vi "ROTPEN Model Validation.vi"() -> ()   [LabVIEW 2018]
uses:
  <vilib>/Simulation/Scripting/Companion Diagram/SimConfigNode/SimParams.ctl
  <vilib>/Simulation/Scripting/Companion Diagram/SimConfigNode/_simSolvers.ctl
  <vilib>/Simulation/Implementation/Shared/SIMSCR Execution Mode.ctl
  <vilib>/Platform/TimedLoop/XDataNode/timing_clust.ctl
  <vilib>/Platform/TimedLoop/XDataNode/nitl_modes.ctl
  <vilib>/Platform/TimedLoop/XDataNode/wakeup.ctl
  <vilib>/Simulation/Param Hierarchy/Typedefs/SIMPH Param Control Actions.ctl
  <vilib>/Simulation/Scripting/Editor Utilities/SIM subVI tag data.ctl
  <vilib>/Simulation/Scripting/Editor Utilities/SIM subVI execution type.ctl
  <vilib>/Simulation/Implementation/Shared/NILVSim_ParamChanged.vi
  <vilib>/Simulation/Implementation/Shared/NILVSim_FinishedLate.vi
  <vilib>/Simulation/Implementation/Shared/NILVSIM_BeginStep.vi
  <vilib>/Simulation/Utility/Implementation/SIM Halt.vi
  <vilib>/Simulation/SignalArithmetic/Implementation/NILVSim Gain.llb/SIM Gain (scalar).vi
  <vilib>/Simulation/ContinuousLinear/Implementation/NILVSim Derivative.llb/SIM derivative (scalar).vi
  <vilib>/Simulation/ContinuousLinear/Implementation/NILVSim Transfer Function.llb/SIM Transfer Function Distributor (SISO).vi
  <vilib>/Simulation/ContinuousLinear/Implementation/NILVSim Transfer Function.llb/SIM Transfer Function Collector (SISO).vi
  <vilib>/Simulation/Implementation/Shared/SIM Fire Discrete SubVI.vi
  <vilib>/Simulation/Implementation/Shared/NILVSim_Manager.vi
  <vilib>/Utility/error.llb/Clear Errors.vi
  <vilib>/Simulation/Implementation/Shared/NILVSim_FinalizeModel.vi
  <vilib>/Simulation/Implementation/Shared/SIM Fire Discrete SubVI (Core).vi
  <vilib>/Simulation/Implementation/Shared/SIM Unbundle Sim Info.vi
  <vilib>/Simulation/Implementation/Shared/SIMSH Read Queue.vi
  <vilib>/Simulation/Implementation/Shared/NILVSim_Initialize.vi
  <vilib>/ptbypt/Signal Generation.llb/Uniform White Noise PtByPt.vi
  <vilib>/Simulation/Utility/Implementation/NILVSim Get Time and IsAcceptedStep.vi
  <vilib>/Simulation/Implementation/Shared/NILVSim_GetModelError.vi
  <vilib>/Simulation/Implementation/Shared/SIM Bundle Sim Info.vi
  <vilib>/Simulation/Scripting/Companion Diagram/SimConfigNode/SimDog.xnode
  <vilib>/Quanser/Rapid Control Prototyping Toolkit/hardware/HIL Immediate IO/_TypeSpecific/CL HIL Read Encoder (Vector).vi
  <vilib>/Quanser/Rapid Control Prototyping Toolkit/hardware/HIL Immediate IO/CL HIL Read.vi
  <vilib>/Platform/TimedLoop/XDataNode/XDataNode.xnode
  <vilib>/Simulation/Implementation/XNodeFramework/SimXNode/SimX.xnode
  <vilib>/Simulation/ContinuousLinear/Implementation/NILVSim Transfer Function.llb/SIM Transfer Function (SISO).vi
  <vilib>/ptbypt/NI_PtbyPt.lvlib
  <vilib>/Platform/TimedLoop/XDataNode/XDNodeRunTimeDep.lvlib
  <vilib>/Simulation/Implementation/Shared/NI_SIM_Implementation.lvlib
panel:
  out "Pendulum Angle  Filter 2":T1(graph)
  out "Hub Angle (deg)":dbl(graph)
  in  "stop":bool
  out "Pendulum Angle (deg)":dbl(graph)
  # "Rotary Hub Angle:  Deg"
  # "Pendulum Angle:  Deg"
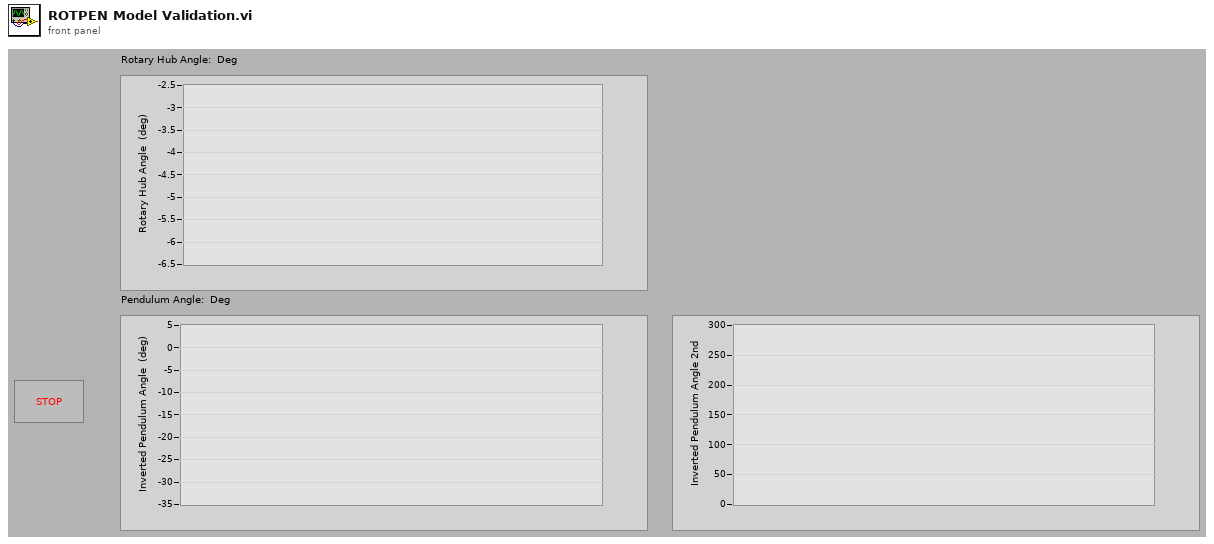
[diagram p1: front panel]
types:
  T1 = cluster{"output":dbl, "output y(t)":dbl, "output y(t)":dbl}
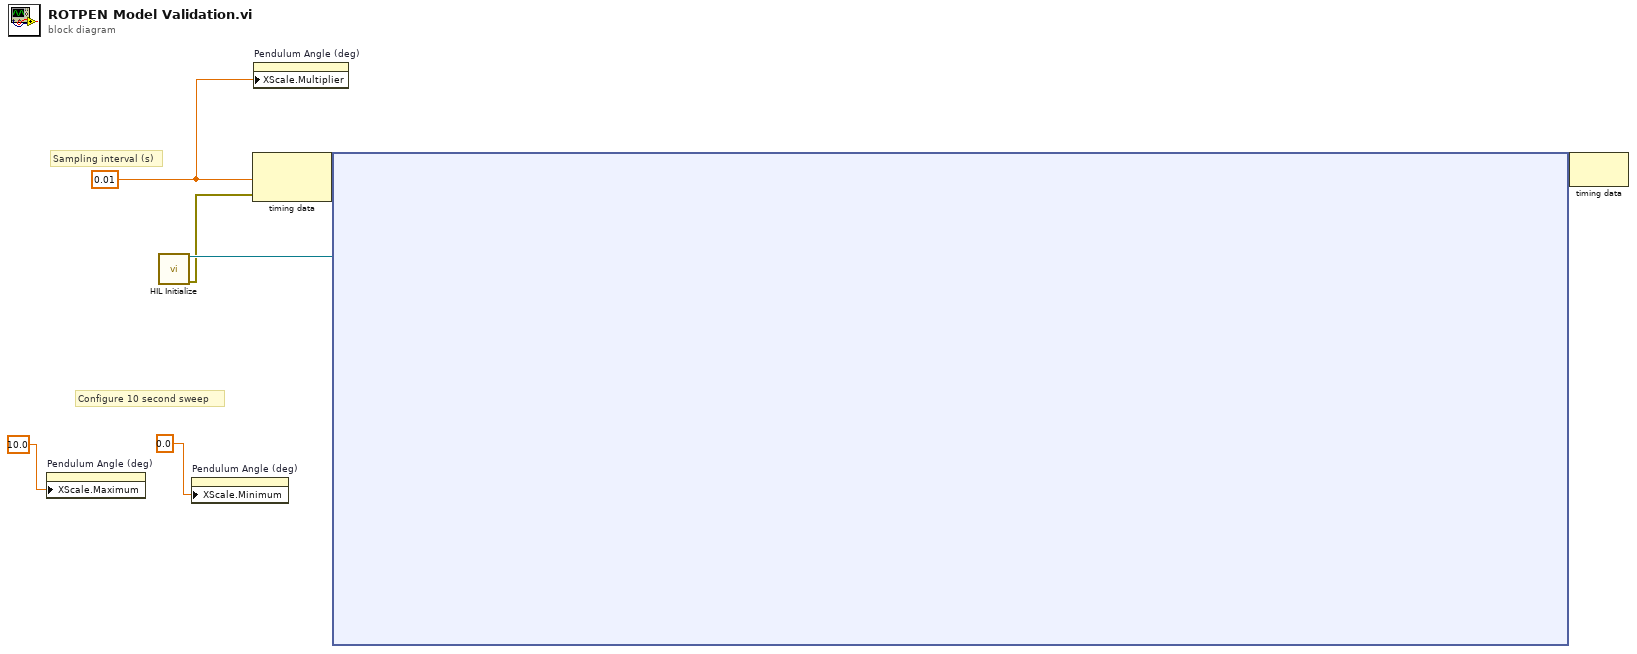
[diagram p0: block diagram]
diagram:
  w3 = 0.01 ("Step Size (s)")
  # "Configure 10 second sweep"
  # "Sampling interval (s)"
  n1 = property on="Pendulum Angle (deg)" class="WFChart (strict)"("XScale.Maximum"=10.0 ("X Scale.Range:Maximum")) -> ()  [unwired: 2 in, 2 out]
  n2 = call "HIL Initialize"() -> ("board out"=w5:refnum<class "HIL Board.lvclass">, "error out"=w4:errorcluster)  [unwired: 14 in]
  n3 = property on="Pendulum Angle (deg)" class="WFChart (strict)"("XScale.Minimum"=0.0 ("X Scale.Range:Maximum")) -> ()  [unwired: 2 in, 2 out]
  n4 = node-c288(w3, w4) -> (w7:variant)
  n5 = property on="Pendulum Angle (deg)" class="WFChart (strict)"("XScale.Multiplier"=w3) -> ()  [unwired: 2 in, 2 out]
  n6 = node-c254 ("Control & Simulation Loop")(w7, w5) -> (w6:variant)
  n7 = node-c288(w6) -> ()  [unwired: 1 out]
